vi "Write error from sender.vi"(8 "error in (no error)":errorcluster, 10 "error from sender":errorcluster, 11 "Report Error Msg in":refnum<class "Report Error Msg Ex.lvclass">) -> (0 "error out":errorcluster, 3 "Report Error Msg out":refnum<class "Report Error Msg Ex.lvclass">)   [LabVIEW 2014, in "Report Error Msg Ex.lvclass"]
uses:
  Report Error Msg Ex.lvclass
  Report Error Msg Ex.lvclass/Report Error Msg Ex.ctl
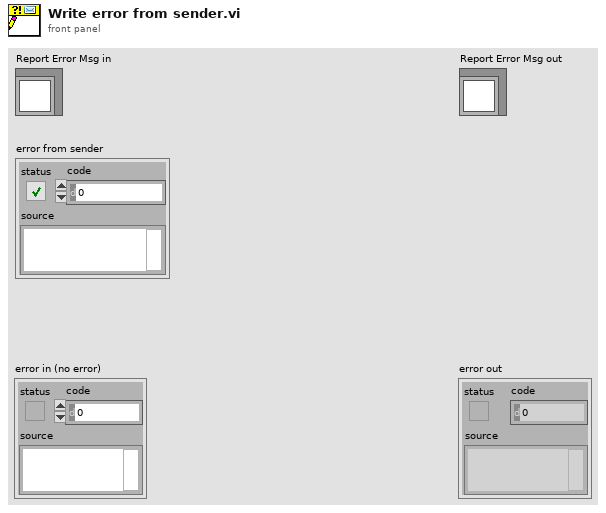
[diagram p1: front panel]
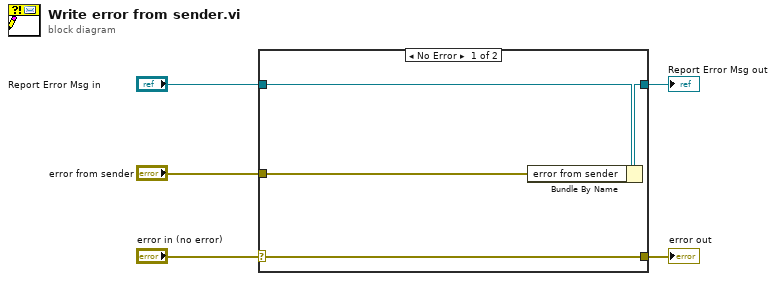
[diagram p0: block diagram]
diagram:
  n1 = case shown="No Error" "error in (no error)" {
    selector: "error in (no error)" -> [w9 w10]
    tunnel: [w9 w10] -> w4
    tunnel: [w7 w11] -> w2
    tunnel: "Report Error Msg in" -> [w8 w11]
    tunnel: "error from sender" -> [w6 _]
    frame No Error {
      n2 = Bundle By Name(cluster=w8, "error from sender"=w6) -> (w7:refnum<class "Report Error Msg Ex.lvclass">)
    }
    frame Error {
    }
  }
  "error out" <- w4
  "Report Error Msg out" <- w2
